vi "Dio3232.vi"(7 "DIO3232_Action":T2, 8 "Error in":errorcluster, 11 "IO In":T1 {"Port" items=["input_port #0", "input_port #1", "input_port #2", "input_port #3", "output_port #0", "output_port #1", "output_port #2", "output_port #3"]}) -> (0 "Error Out":errorcluster, 3 "IO Out":T1 {"Port" items=["input_port #0", "input_port #1", "input_port #2", "input_port #3", "output_port #0", "output_port #1", "output_port #2", "output_port #3"]})   [LabVIEW 2015]
uses:
  Main_IO_3232.ctl
  Dio3232_controls.ctl
panel:
  # "input_port0  ÂI¦ìinput0~7\ninput_port1  ÂI¦ìinput8~15\ninput_port2  ÂI¦ìinput16~23\ninput_port3  ÂI¦ìinput24~31"
  # "output_port0  ÂI¦ìoutput0~7\noutput_port1  ÂI¦ìoutput8~15\noutput_port2  ÂI¦ìoutput16~23\noutput_port3  ÂI¦ìoutput24~31"
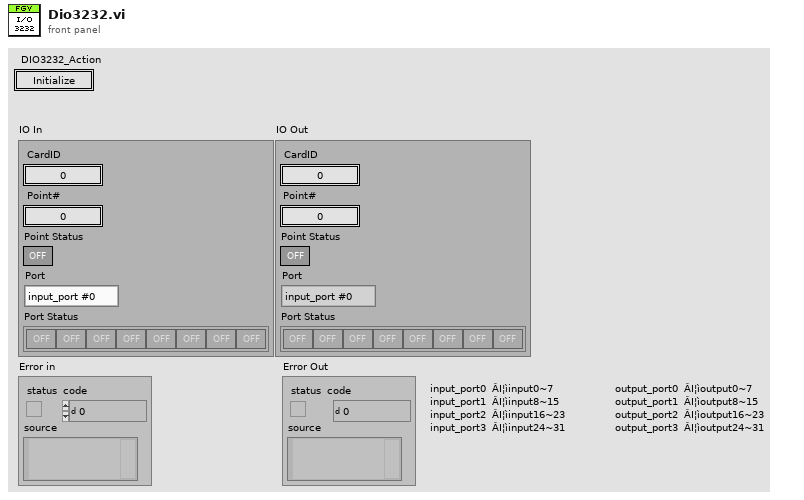
[diagram p1: front panel]
types:
  T1 = typedef "Main_IO_3232.ctl" = cluster{"CardID":u8, "Point#":u8, "Point Status":bool, "Port Status":bool[], "Port":u8}
  T2 = typedef "Dio3232_controls.ctl" = enum16{"Initialize", "Set Point", "Set Port", "Read In Point", "Read Out Point", "Read Port", "Close", "Idle"}
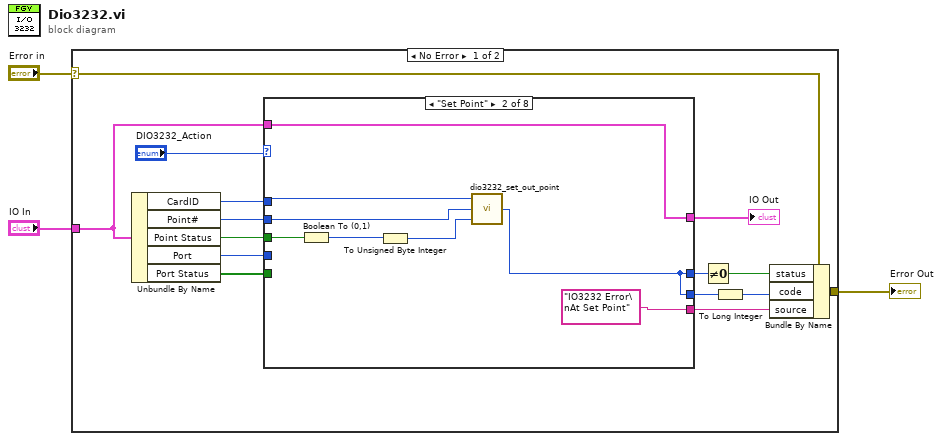
[diagram p0: block diagram]
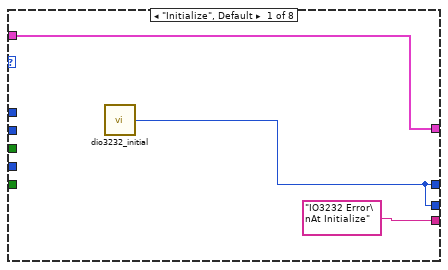
[diagram p2: hidden frame]
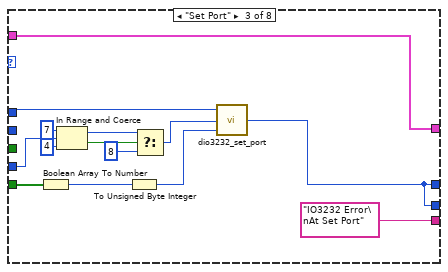
[diagram p3: hidden frame]
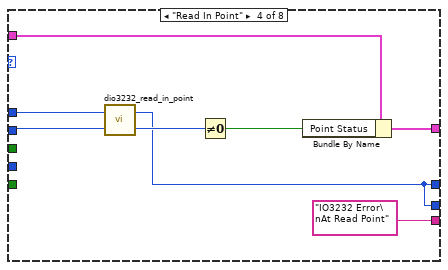
[diagram p4: hidden frame]
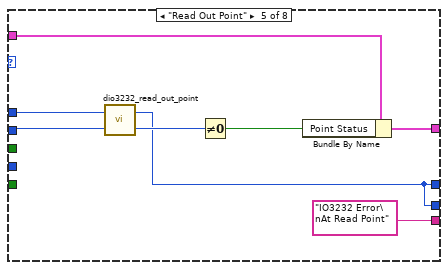
[diagram p5: hidden frame]
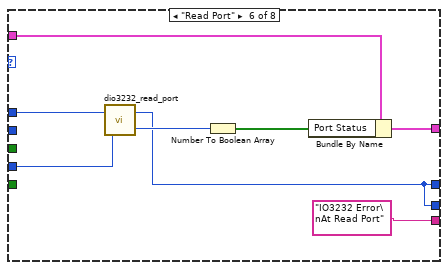
[diagram p6: hidden frame]
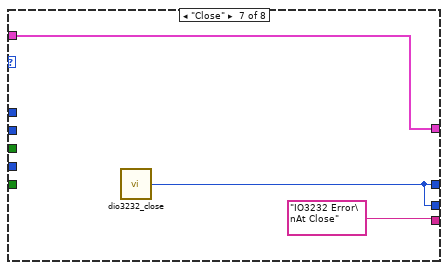
[diagram p7: hidden frame]
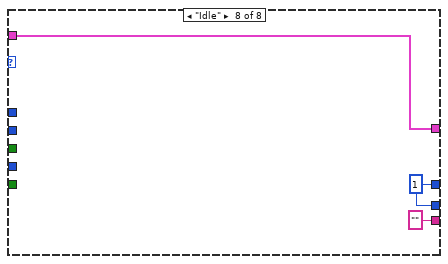
[diagram p8: hidden frame]
diagram:
  n1 = case shown="No Error" "Error in" {
    selector: "Error in" -> [w8 w74]
    tunnel: "IO In" -> [w13 _]
    tunnel: [w11 w74] -> w2
    frame No Error {
      n2 = Unbundle By Name(w13) -> ("CardID"=w18:u8, "Point#"=w17:u8, "Point Status"=w15:bool, "Port"=w16:u8, "Port Status"=w14:bool[])
      n3 = case shown="\"Set Point\"" "DIO3232_Action" {
        tunnel: w18 -> [_ w25 w39 w47 w55 w63 _ _]
        tunnel: w17 -> [_ w24 _ w46 w54 _ _ _]
        tunnel: w15 -> [_ w29 _ _ _ _ _ _]
        tunnel: w16 -> [_ _ w31 _ _ w62 _ _]
        tunnel: w14 -> [_ _ w43 _ _ _ _ _]
        tunnel: w13 -> [w21 w27 w41 w51 w58 w66 w70 w73]
        tunnel: [w21 w27 w41 w50 w57 w67 w70 w73] -> w7
        tunnel: [w19 w22 w37 w44 w52 w60 w68 w71] -> w12
        tunnel: ["IO3232 Error\nAt Initialize" "IO3232 Error\nAt Set Point" "IO3232 Error\nAt Set Port" "IO3232 Error\nAt Read Point" "IO3232 Error\nAt Read Point" "IO3232 Error\nAt Read Port" "IO3232 Error\nAt Close" ""] -> w9
        tunnel: [w19 w22 w37 w44 w52 w60 w68 w71] -> w4
        frame "Initialize", Default {
          n4 = call <vilib>:"dio3232_initial.vi"() -> ("error_code"=w19:u32)
        }
        frame "Set Point" {
          n5 = Boolean To (0,1)(Boolean=w29) -> (0, 1=w28:i16)
          n6 = To Unsigned Byte Integer(number=w28) -> (unsigned 8bit integer=w23:u8)
          n7 = call <vilib>:"dio3232_set_out_point.vi"("State"=w23, "Point"=w24, "CardID"=w25) -> ("error_code"=w22:u32)
        }
        frame "Set Port" {
          n8 = Boolean Array To Number(Boolean array=w43) -> (number=w42:u32)
          n9 = In Range and Coerce(upper limit=u8 7, x=w31, lower limit=u8 4) -> (coerced(x)=w36:u8, In Range?=w34:bool)
          n10 = To Unsigned Byte Integer(number=w42) -> (unsigned 8bit integer=w38:u8)
          n11 = Select(t=w36, s=w34, f=u8 8) -> (s? t:f=w30:u8)
          n12 = call <vilib>:"dio3232_set_port.vi"("Data"=w38, "Port"=w30, "CardID"=w39) -> ("error_code"=w37:u32)
        }
        frame "Read In Point" {
          n13 = call <vilib>:"dio3232_read_in_point.vi"("Point"=w46, "CardID"=w47) -> ("State"=w45:u8, "error_code"=w44:u32)
          n14 = Not Equal To 0?(x=w45) -> (x != 0?=w49:bool)
          n15 = Bundle By Name(cluster=w51, "Point Status"=w49) -> (w50:T1)
        }
        frame "Read Out Point" {
          n16 = call <vilib>:"dio3232_read_out_point.vi"("Point"=w54, "CardID"=w55) -> ("State"=w53:u8, "error_code"=w52:u32)
          n17 = Not Equal To 0?(x=w53) -> (x != 0?=w59:bool)
          n18 = Bundle By Name(cluster=w58, "Point Status"=w59) -> (w57:T1)
        }
        frame "Read Port" {
          n19 = call <vilib>:"dio3232_read_port.vi"("Port"=w62, "CardID"=w63) -> ("Data"=w61:u8, "error_code"=w60:u32)
          n20 = Number To Boolean Array(number=w61) -> (Boolean array=w65:bool[])
          n21 = Bundle By Name(cluster=w66, "Port Status"=w65) -> (w67:T1)
        }
        frame "Close" {
          n22 = call <vilib>:"dio3232_close.vi"() -> ("error_code"=w68:u32)
        }
        frame "Idle" {
          w71 = u32 1 ("error_code")
        }
      }
      "IO Out" <- w7
      n23 = Not Equal To 0?(x=w12) -> (x != 0?=w10:bool)
      n24 = To Long Integer(number=w4) -> (32bit integer=w5:i32)
      n25 = Bundle By Name(cluster=w8, "status"=w10, "code"=w5, "source"=w9) -> (w11:errorcluster)
    }
    frame Error {
    }
  }
  "Error Out" <- w2
